vi "Write software version.vi"(8 "error in (no error)":errorcluster, 11 "Channel in":refnum<class "Channel.lvclass">) -> (0 "error out":errorcluster, 2 "ACS version":string, 3 "Channel out":refnum<class "Channel.lvclass">)   [LabVIEW 2018, in "Channel.lvclass"]
uses:
  Channel.lvclass
  Channel.lvclass/Channel.ctl
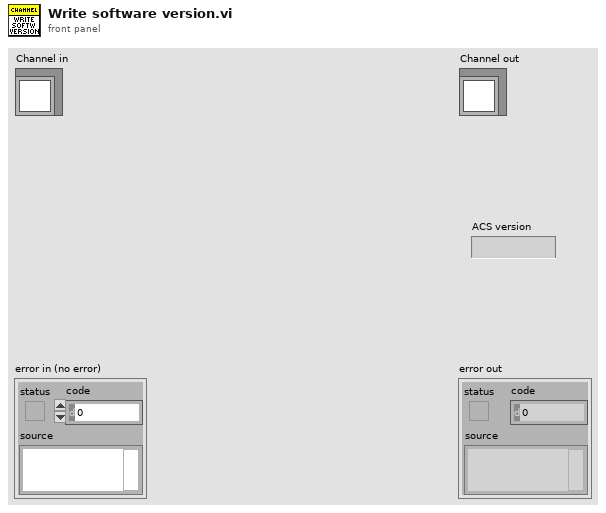
[diagram p1: front panel]
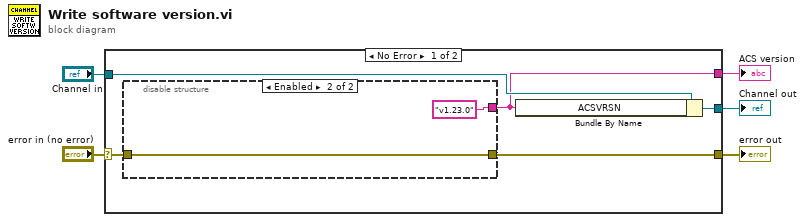
[diagram p0: block diagram]
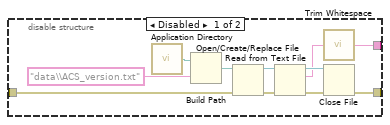
[diagram p2: hidden frame]
diagram:
  n1 = case shown="No Error" "error in (no error)" {
    selector: "error in (no error)" -> [w9 w25]
    tunnel: [w10 w25] -> w4
    tunnel: [w7 w24] -> w2
    tunnel: "Channel in" -> [w8 w24]
    tunnel: [w6 _] -> w1
    frame No Error {
      n2 = disable-structure shown="Enabled" {
        disable-tunnel: [w21 w23] -> w10
        disable-tunnel: w9 -> [w20 w23]
        disable-tunnel: [w11 "v1.23.0" ("trimmed string")] -> w6
        frame Disabled {
          n3 = call <vilib>:"Application Directory.vi"() -> ("Application Directory"=w14:path)
          n4 = Build Path(base path=w14, name or relative path="data\\ACS_version.txt") -> (appended path=w15:path)
          n5 = Open/Create/Replace File(file path (use dialog)=w15, error in=w20) -> (refnum out=w19:refnum<file>, error out=w18:errorcluster)  [unwired: 4 in, 1 out]
          n6 = Read from Text File(file (use dialog)=w19, error in=w18) -> (refnum out=w16:refnum<file>, text=w12:string, error out=w17:errorcluster)  [unwired: 2 in, 1 out]
          n7 = call <vilib>:"Trim Whitespace.vi"("string"=w12) -> ("trimmed string"=w11:string)  [unwired: 1 in]
          n8 = Close File(refnum=w16, error in=w17) -> (error out=w21:errorcluster)  [unwired: 1 out]
        }
        frame Enabled {
        }
      }
      n9 = Bundle By Name(cluster=w8, "ACSVRSN"=w6) -> (w7:refnum<class "Channel.lvclass">)
    }
    frame Error {
    }
  }
  "error out" <- w4
  "Channel out" <- w2
  "ACS version" <- w1
